vi "map_XY_stiffback.vi"() -> ()   [LabVIEW 2011]
panel:
  in  "KILL":bool
  in  "PAUSE":bool
  in  "RESUME":bool
  in  "QUIT":bool
  in  "up done":bool
  in  "z up":bool
  in  "Done":bool
  in  "z go to table 2":bool
  in  "z go to table":bool
  in  "go to y pos":bool
  in  "goto x pos":bool
  in  "End":bool
  in  "zero z - end":bool
  in  "zero x - end":bool
  in  "zero y - end":bool
  in  "goto z pos":bool
  in  "positioning done":bool
  out "output":string
  out "command":string
  in  "zero done":bool
  in  "zero z":bool
  in  "zero x":bool
  in  "zero y":bool
  # "Comandi di emergenza"
  # "MAPPING XY STIFFBACK"
  # "Posiziono in zero"
  # "Vado sulla piastra \ne azzero"
  # "Alzo il comparatore"
  # "Vado in posizione"
  # "Ritorno a zero"
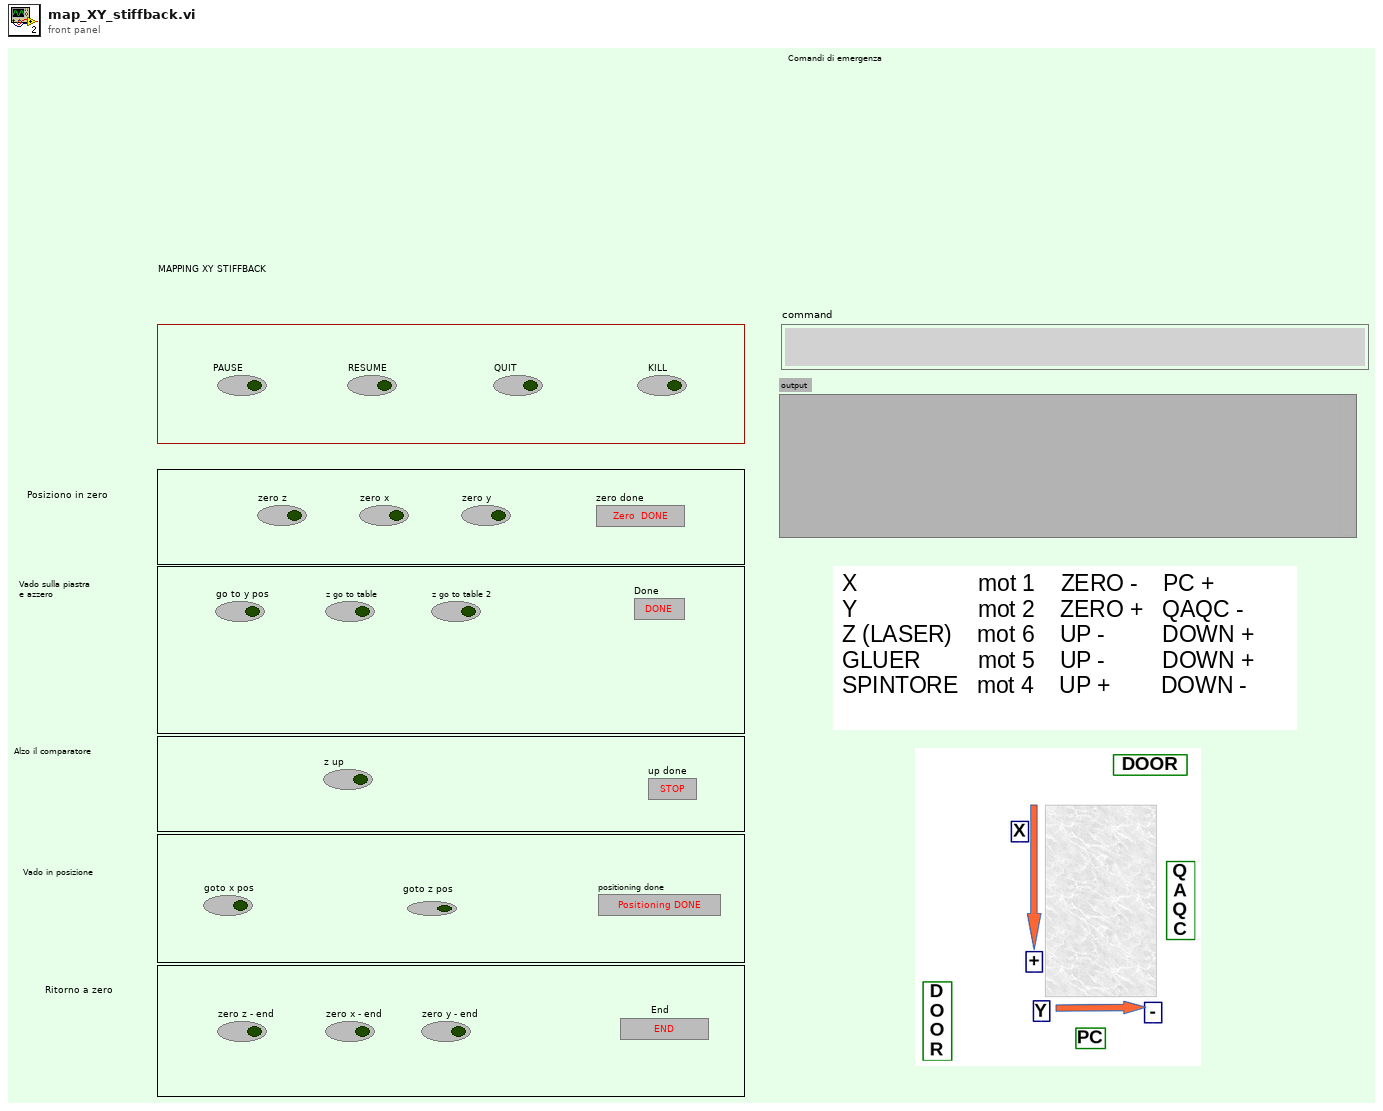
[diagram p1: front panel]
types:
  T1 = enum16{"open", "replace", "create", "open or create", "replace or create", "replace or create with confirmation"}
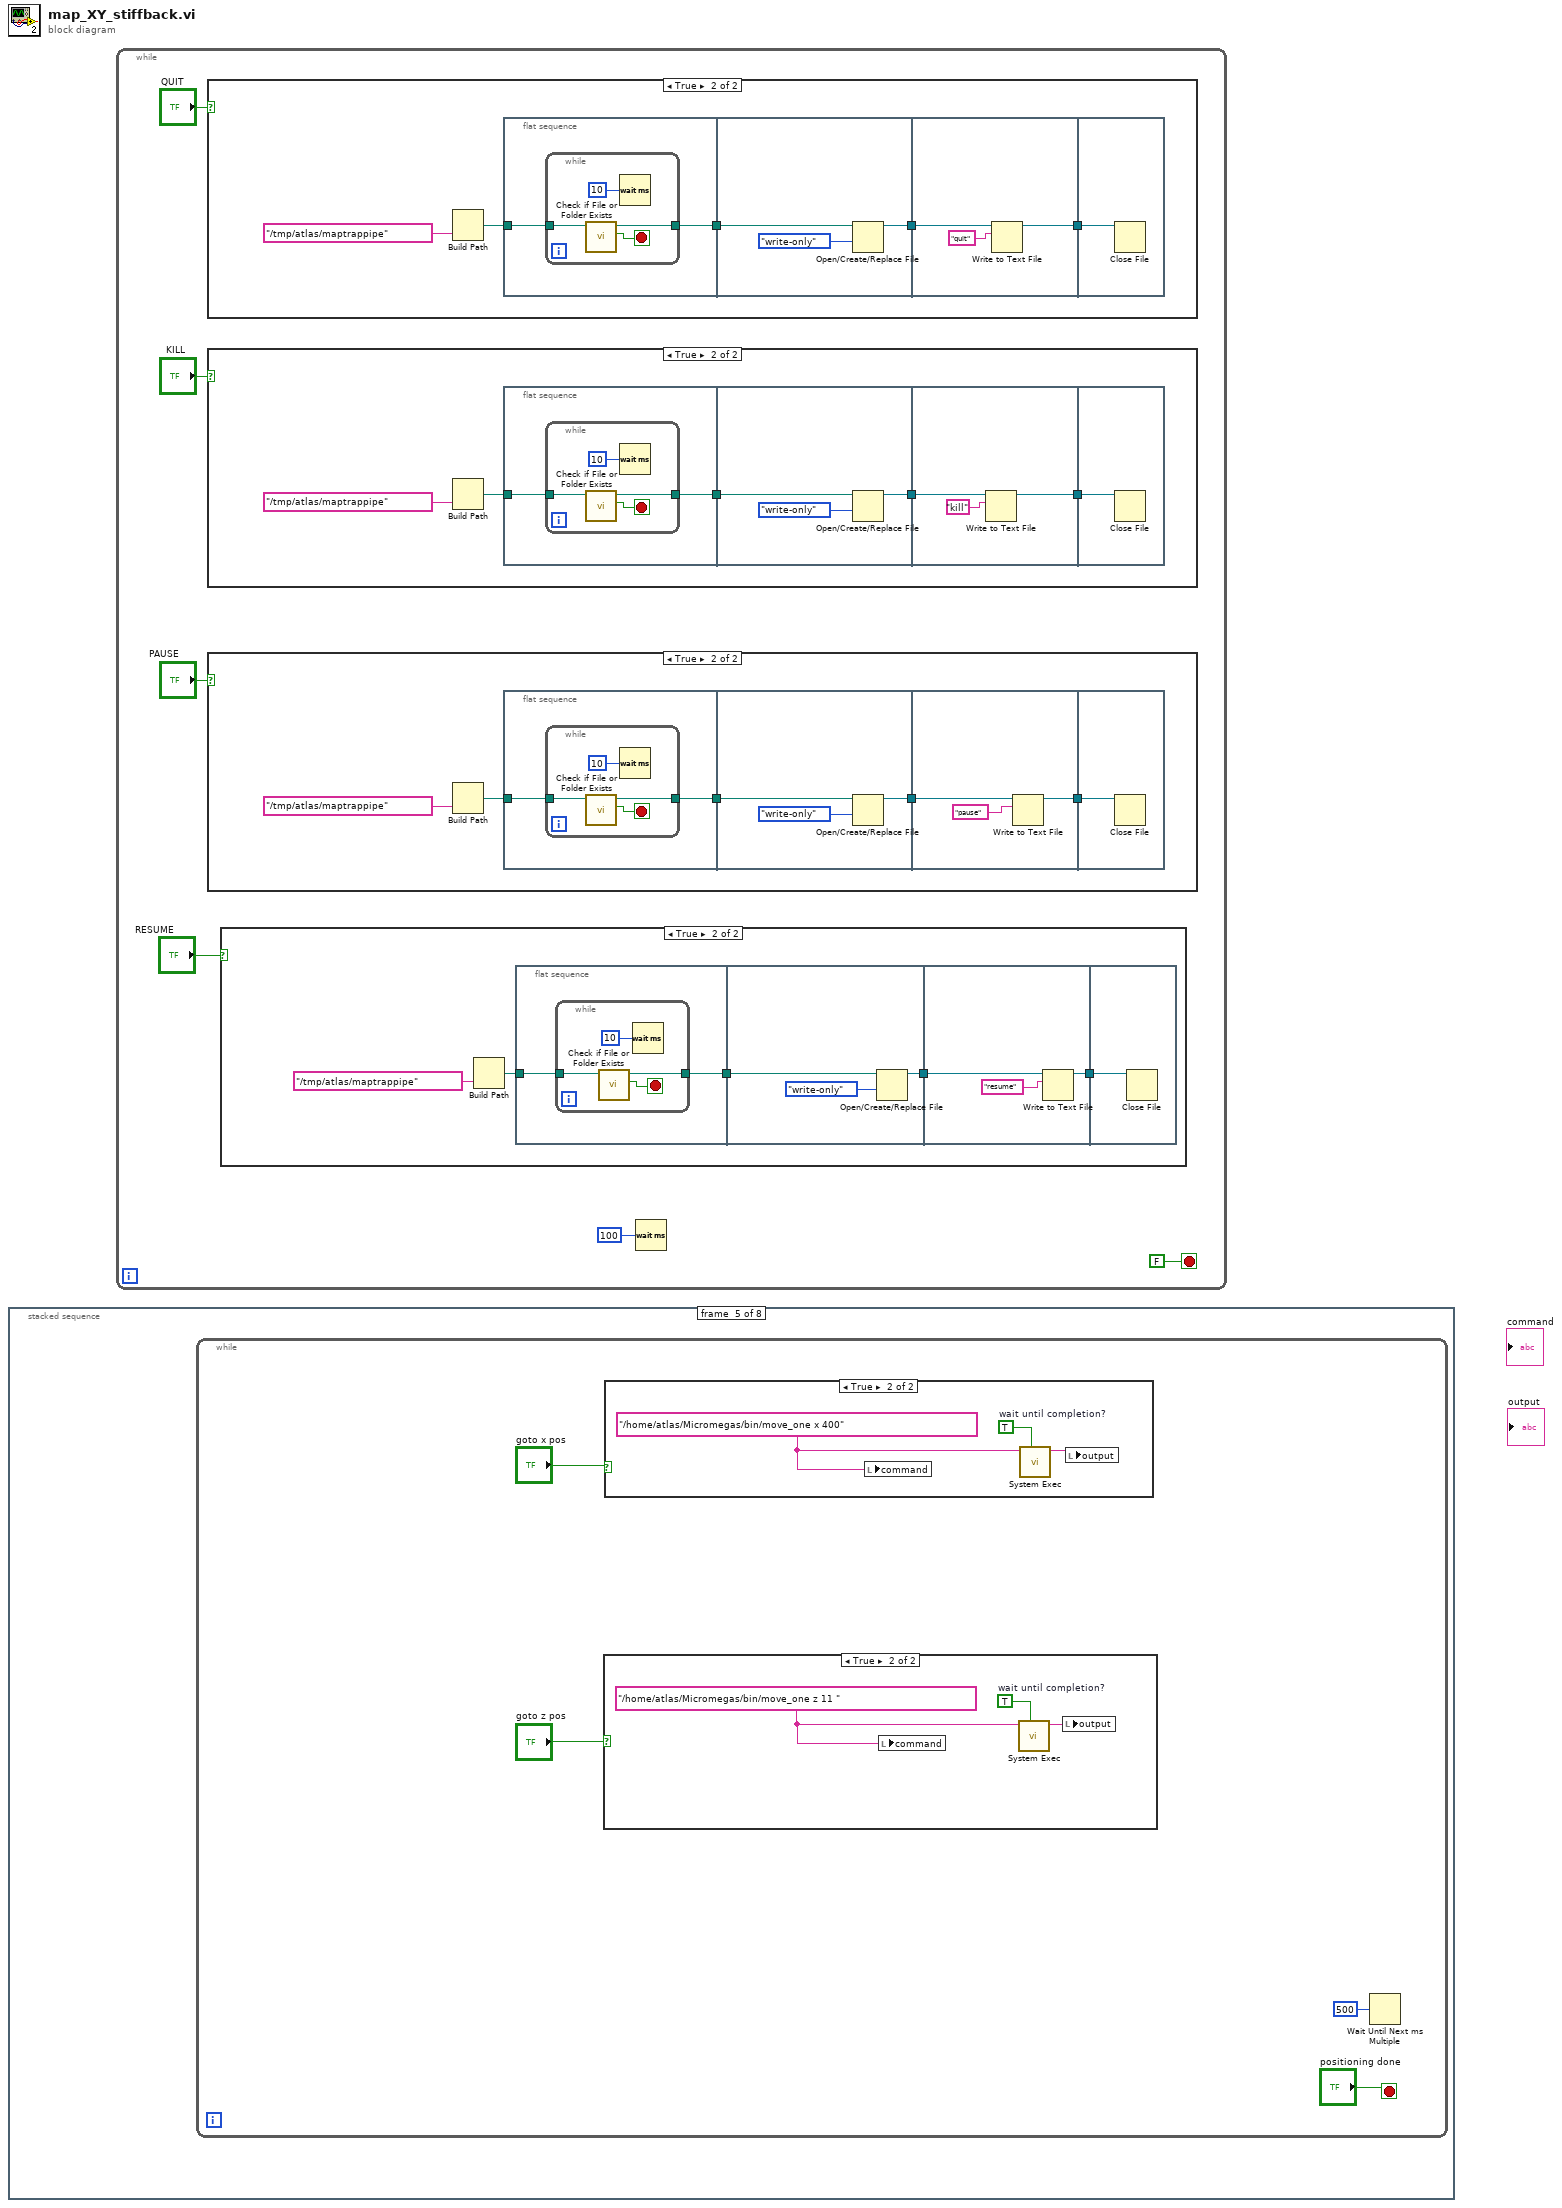
[diagram p0: block diagram]
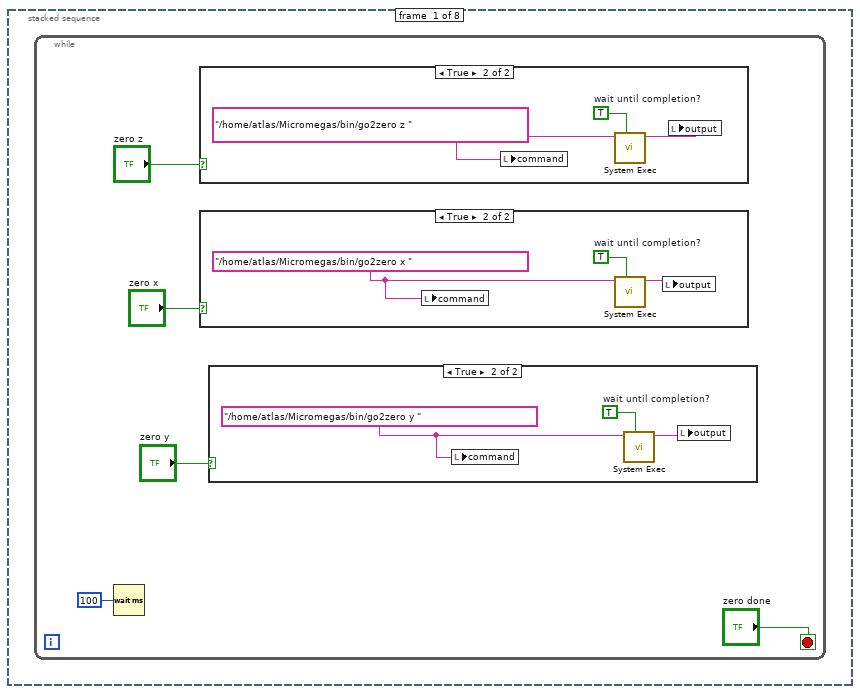
[diagram p6: hidden frame]
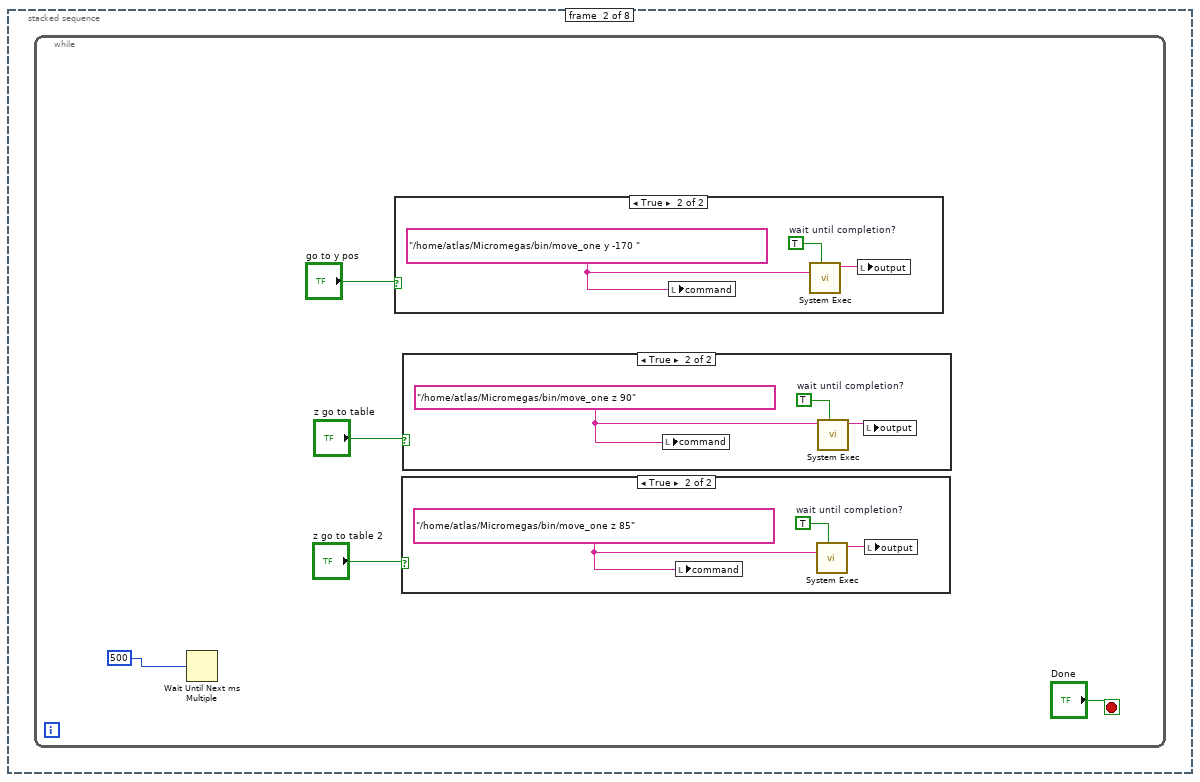
[diagram p10: hidden frame]
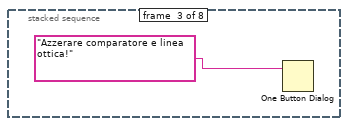
[diagram p14: hidden frame]
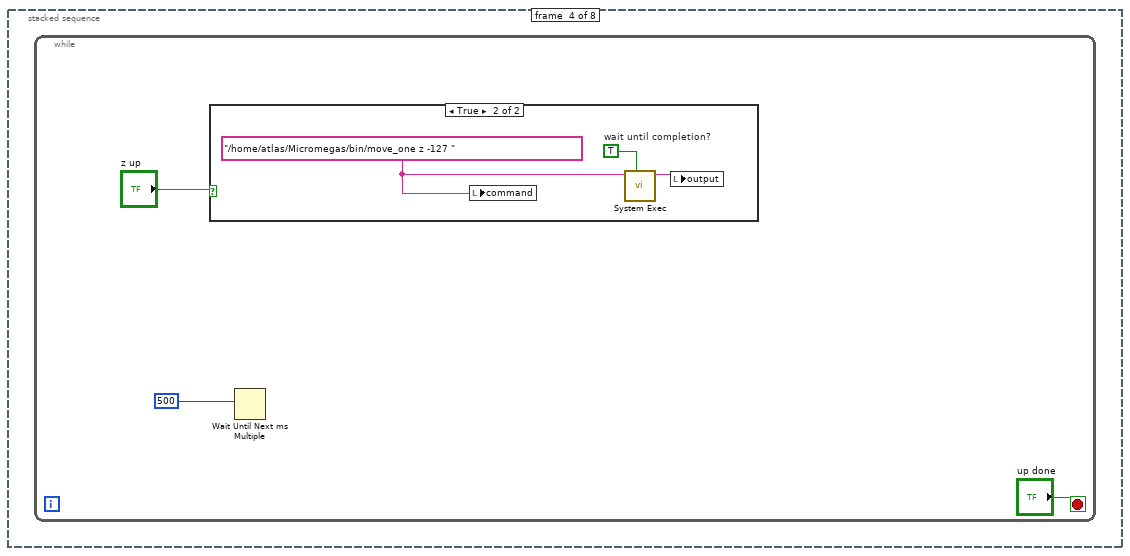
[diagram p15: hidden frame]
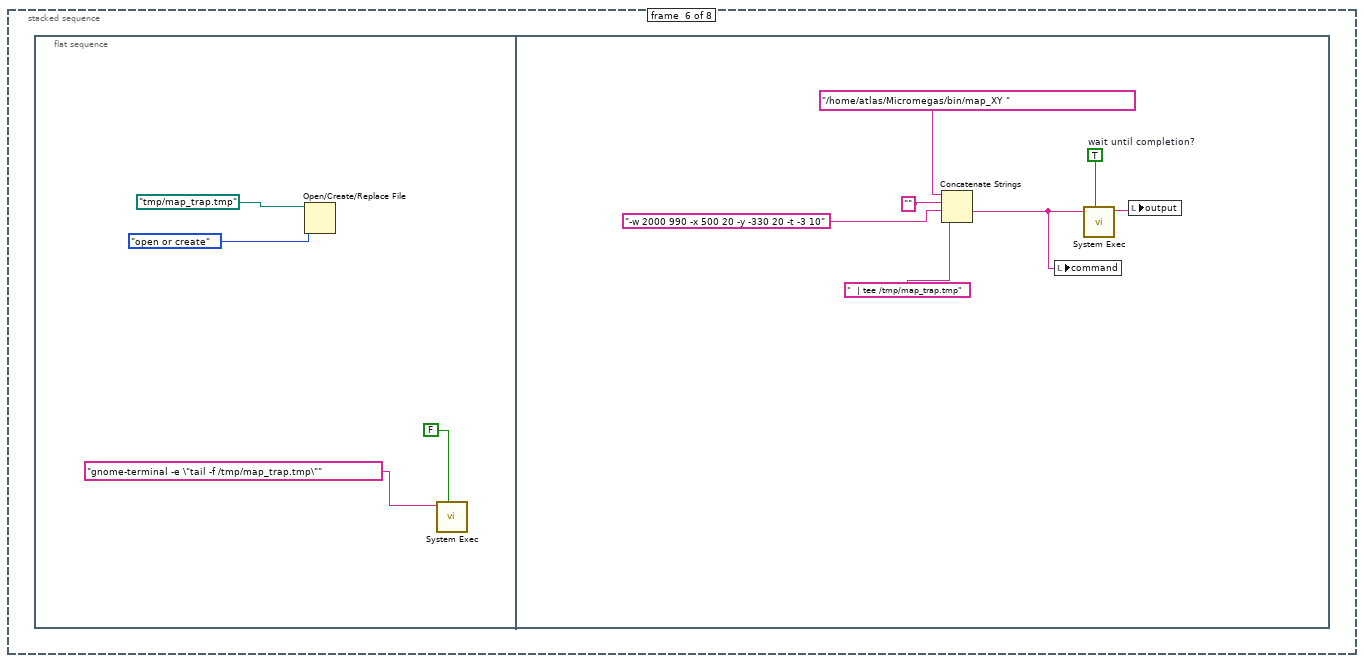
[diagram p19: hidden frame]
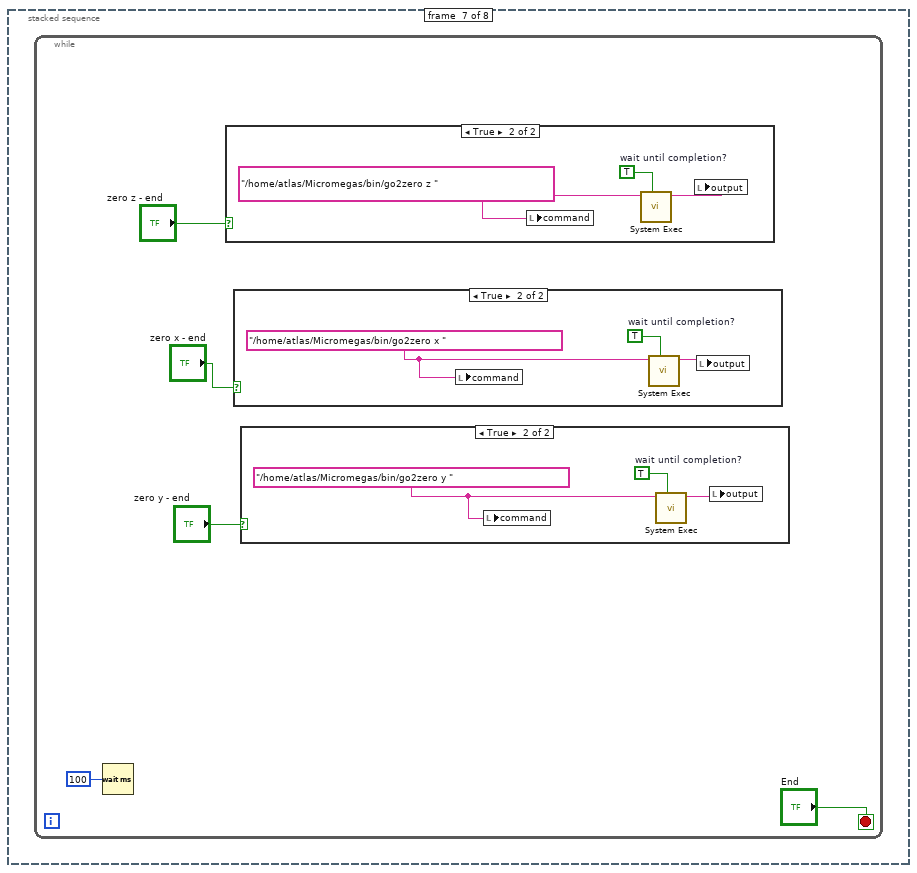
[diagram p20: hidden frame]
diagram:
  n1 = stacked-sequence {
    frame #0 {
      n2 = while {
        stop <- "zero done" stop-if-true
        n3 = Wait (ms)(milliseconds to wait=u32 100) -> ()  [unwired: 1 out]
        n4 = case shown="True" "zero z" {
          frame False {
          }
          frame True {
            w13 = "/home/atlas/Micromegas/bin/go2zero z " ("string")
            w14 = TRUE  # wait until completion?
            n5 = local write "command"(w13) -> ()
            n6 = call <vilib>:"System Exec.vi"("wait until completion? (T)"=w14, "command line"=w13) -> ("standard output"=w12:string)  [unwired: 6 in, 3 out]
            n7 = local write "output"(w12) -> ()
          }
        }
        n8 = case shown="True" "zero x" {
          frame False {
          }
          frame True {
            w10 = "/home/atlas/Micromegas/bin/go2zero x " ("string")
            w11 = TRUE  # wait until completion?
            n9 = local write "command"(w10) -> ()
            n10 = call <vilib>:"System Exec.vi"("wait until completion? (T)"=w11, "command line"=w10) -> ("standard output"=w9:string)  [unwired: 6 in, 3 out]
            n11 = local write "output"(w9) -> ()
          }
        }
        n12 = case shown="True" "zero y" {
          frame False {
          }
          frame True {
            w7 = "/home/atlas/Micromegas/bin/go2zero y " ("string")
            w8 = TRUE  # wait until completion?
            n13 = local write "command"(w7) -> ()
            n14 = call <vilib>:"System Exec.vi"("wait until completion? (T)"=w8, "command line"=w7) -> ("standard output"=w6:string)  [unwired: 6 in, 3 out]
            n15 = local write "output"(w6) -> ()
          }
        }
      }
    }
    frame #1 {
      n16 = while {
        stop <- "Done" stop-if-true
        n17 = Wait Until Next ms Multiple(millisecond multiple=u32 500 ("millisecond timer value")) -> ()  [unwired: 1 out]
        n18 = case shown="True" "go to y pos" {
          frame False {
          }
          frame True {
            w26 = "/home/atlas/Micromegas/bin/move_one y -170 " ("string")
            w28 = TRUE  # wait until completion?
            n19 = local write "command"(w26) -> ()
            n20 = call <vilib>:"System Exec.vi"("wait until completion? (T)"=w28, "command line"=w26) -> ("standard output"=w27:string)  [unwired: 6 in, 3 out]
            n21 = local write "output"(w27) -> ()
          }
        }
        n22 = case shown="True" "z go to table 2" {
          frame False {
          }
          frame True {
            w20 = "/home/atlas/Micromegas/bin/move_one z 85" ("string")
            w22 = TRUE  # wait until completion?
            n23 = local write "command"(w20) -> ()
            n24 = call <vilib>:"System Exec.vi"("wait until completion? (T)"=w22, "command line"=w20) -> ("standard output"=w21:string)  [unwired: 6 in, 3 out]
            n25 = local write "output"(w21) -> ()
          }
        }
        n26 = case shown="True" "z go to table" {
          frame False {
          }
          frame True {
            w23 = "/home/atlas/Micromegas/bin/move_one z 90" ("string")
            w25 = TRUE  # wait until completion?
            n27 = local write "command"(w23) -> ()
            n28 = call <vilib>:"System Exec.vi"("wait until completion? (T)"=w25, "command line"=w23) -> ("standard output"=w24:string)  [unwired: 6 in, 3 out]
            n29 = local write "output"(w24) -> ()
          }
        }
      }
    }
    frame #2 {
      n30 = One Button Dialog(message="Azzerare comparatore e linea ottica!") -> ()  [unwired: 1 in, 1 out]
    }
    frame #3 {
      n31 = while {
        stop <- "up done" stop-if-true
        n32 = case shown="True" "z up" {
          frame False {
          }
          frame True {
            w33 = "/home/atlas/Micromegas/bin/move_one z -127 " ("string")
            w35 = TRUE  # wait until completion?
            n33 = local write "command"(w33) -> ()
            n34 = call <vilib>:"System Exec.vi"("wait until completion? (T)"=w35, "command line"=w33) -> ("standard output"=w34:string)  [unwired: 6 in, 3 out]
            n35 = local write "output"(w34) -> ()
          }
        }
        n36 = Wait Until Next ms Multiple(millisecond multiple=u32 500 ("millisecond timer value")) -> ()  [unwired: 1 out]
      }
    }
    frame #4 {
      n37 = while {
        stop <- "positioning done" stop-if-true
        n38 = case shown="True" "goto z pos" {
          frame False {
          }
          frame True {
            w40 = "/home/atlas/Micromegas/bin/move_one z 11 " ("string")
            w42 = TRUE  # wait until completion?
            n39 = local write "command"(w40) -> ()
            n40 = call <vilib>:"System Exec.vi"("wait until completion? (T)"=w42, "command line"=w40) -> ("standard output"=w41:string)  [unwired: 6 in, 3 out]
            n41 = local write "output"(w41) -> ()
          }
        }
        n42 = case shown="True" "goto x pos" {
          frame False {
          }
          frame True {
            w43 = "/home/atlas/Micromegas/bin/move_one x 400" ("string")
            w45 = TRUE  # wait until completion?
            n43 = local write "command"(w43) -> ()
            n44 = call <vilib>:"System Exec.vi"("wait until completion? (T)"=w45, "command line"=w43) -> ("standard output"=w44:string)  [unwired: 6 in, 3 out]
            n45 = local write "output"(w44) -> ()
          }
        }
        n46 = Wait Until Next ms Multiple(millisecond multiple=u32 500) -> ()  [unwired: 1 out]
      }
    }
    frame #5 {
      n47 = flat-sequence {
        frame #0 {
          n48 = Open/Create/Replace File(file path (use dialog)=path "/tmp/map_trap.tmp", operation (0:open)=T1."open or create") -> ()  [unwired: 4 in, 3 out]
          n49 = call <vilib>:"System Exec.vi"("wait until completion? (T)"=FALSE, "command line"="gnome-terminal -e \"tail -f /tmp/map_trap.tmp\"") -> ()  [unwired: 6 in, 4 out]
        }
        frame #1 {
          w56 = TRUE  # wait until completion?
          n50 = Concatenate Strings("/home/atlas/Micromegas/bin/map_XY " ("string"), "" ("string"), "-w 2000 990 -x 500 20 -y -330 20 -t -3 10" ("string"), "  | tee /tmp/map_trap.tmp" ("string")) -> (w51:string)
          n51 = local write "command"(w51) -> ()
          n52 = call <vilib>:"System Exec.vi"("wait until completion? (T)"=w56, "command line"=w51) -> ("standard output"=w50:string)  [unwired: 6 in, 3 out]
          n53 = local write "output"(w50) -> ()
        }
      }
    }
    frame #6 {
      n54 = while {
        stop <- "End" stop-if-true
        n55 = Wait (ms)(milliseconds to wait=u32 100) -> ()  [unwired: 1 out]
        n56 = case shown="True" "zero z - end" {
          frame False {
          }
          frame True {
            w69 = "/home/atlas/Micromegas/bin/go2zero z " ("string")
            w70 = TRUE  # wait until completion?
            n57 = local write "command"(w69) -> ()
            n58 = call <vilib>:"System Exec.vi"("wait until completion? (T)"=w70, "command line"=w69) -> ("standard output"=w68:string)  [unwired: 6 in, 3 out]
            n59 = local write "output"(w68) -> ()
          }
        }
        n60 = case shown="True" "zero x - end" {
          frame False {
          }
          frame True {
            w66 = "/home/atlas/Micromegas/bin/go2zero x " ("string")
            w67 = TRUE  # wait until completion?
            n61 = local write "command"(w66) -> ()
            n62 = call <vilib>:"System Exec.vi"("wait until completion? (T)"=w67, "command line"=w66) -> ("standard output"=w65:string)  [unwired: 6 in, 3 out]
            n63 = local write "output"(w65) -> ()
          }
        }
        n64 = case shown="True" "zero y - end" {
          frame False {
          }
          frame True {
            w63 = "/home/atlas/Micromegas/bin/go2zero y " ("string")
            w64 = TRUE  # wait until completion?
            n65 = local write "command"(w63) -> ()
            n66 = call <vilib>:"System Exec.vi"("wait until completion? (T)"=w64, "command line"=w63) -> ("standard output"=w62:string)  [unwired: 6 in, 3 out]
            n67 = local write "output"(w62) -> ()
          }
        }
      }
    }
    frame #7 {
      n68 = One Button Dialog(message="Per comodita`, rinominare il file (non verra` comunque sovrascritto)") -> ()  [unwired: 1 in, 1 out]
    }
  }
  n69 = while {
    stop <- FALSE stop-if-true
    n70 = case shown="True" "QUIT" {
      frame False {
      }
      frame True {
        n71 = Build Path(name or relative path="/tmp/atlas/maptrappipe" ("string")) -> (appended path=w132:path)  [unwired: 1 in]
        n72 = flat-sequence {
          tunnel: [w138] -> w136
          tunnel: w132 -> [w137]
          tunnel: w136 -> [w145]
          tunnel: [w143] -> w135
          tunnel: w135 -> [w148]
          tunnel: [w147] -> w134
          tunnel: w134 -> [w149]
          frame #0 {
            n73 = while {
              tunnel: [w140] -> w138
              tunnel: w137 -> [w139]
              stop <- w141 stop-if-true
              n74 = call <vilib>:"Check if File or Folder Exists.vi"("path"=w139) -> ("file or folder exists?"=w141:bool, "dup path"=w140:path)  [unwired: 8 in, 1 out]
              n75 = Wait (ms)(milliseconds to wait=u32 10) -> ()  [unwired: 1 out]
            }
          }
          frame #1 {
            n76 = Open/Create/Replace File(file path (use dialog)=w145, access (0:read/write)=enum16{"read/write", "read-only", "write-only"}."write-only") -> (refnum out=w143:refnum<file>)  [unwired: 4 in, 2 out]
          }
          frame #2 {
            n77 = Write to Text File(file (use dialog)=w148, text="quit") -> (refnum out=w147:refnum<file>)  [unwired: 2 in, 2 out]
          }
          frame #3 {
            n78 = Close File(refnum=w149) -> ()  [unwired: 1 in, 2 out]
          }
        }
      }
    }
    n79 = case shown="True" "KILL" {
      frame False {
      }
      frame True {
        n80 = Build Path(name or relative path="/tmp/atlas/maptrappipe" ("string")) -> (appended path=w96:path)  [unwired: 1 in]
        n81 = flat-sequence {
          tunnel: [w102] -> w100
          tunnel: w96 -> [w101]
          tunnel: w100 -> [w109]
          tunnel: [w107] -> w99
          tunnel: w99 -> [w112]
          tunnel: [w111] -> w98
          tunnel: w98 -> [w113]
          frame #0 {
            n82 = while {
              tunnel: [w104] -> w102
              tunnel: w101 -> [w103]
              stop <- w105 stop-if-true
              n83 = call <vilib>:"Check if File or Folder Exists.vi"("path"=w103) -> ("file or folder exists?"=w105:bool, "dup path"=w104:path)  [unwired: 8 in, 1 out]
              n84 = Wait (ms)(milliseconds to wait=u32 10) -> ()  [unwired: 1 out]
            }
          }
          frame #1 {
            n85 = Open/Create/Replace File(file path (use dialog)=w109, access (0:read/write)=enum16{"read/write", "read-only", "write-only"}."write-only") -> (refnum out=w107:refnum<file>)  [unwired: 4 in, 2 out]
          }
          frame #2 {
            n86 = Write to Text File(file (use dialog)=w112, text="kill") -> (refnum out=w111:refnum<file>)  [unwired: 2 in, 2 out]
          }
          frame #3 {
            n87 = Close File(refnum=w113) -> ()  [unwired: 1 in, 2 out]
          }
        }
      }
    }
    n88 = case shown="True" "PAUSE" {
      frame False {
      }
      frame True {
        n89 = Build Path(name or relative path="/tmp/atlas/maptrappipe" ("string")) -> (appended path=w78:path)  [unwired: 1 in]
        n90 = flat-sequence {
          tunnel: [w84] -> w82
          tunnel: w78 -> [w83]
          tunnel: w82 -> [w91]
          tunnel: [w89] -> w81
          tunnel: w81 -> [w94]
          tunnel: [w93] -> w80
          tunnel: w80 -> [w95]
          frame #0 {
            n91 = while {
              tunnel: [w86] -> w84
              tunnel: w83 -> [w85]
              stop <- w87 stop-if-true
              n92 = call <vilib>:"Check if File or Folder Exists.vi"("path"=w85) -> ("file or folder exists?"=w87:bool, "dup path"=w86:path)  [unwired: 8 in, 1 out]
              n93 = Wait (ms)(milliseconds to wait=u32 10) -> ()  [unwired: 1 out]
            }
          }
          frame #1 {
            n94 = Open/Create/Replace File(file path (use dialog)=w91, access (0:read/write)=enum16{"read/write", "read-only", "write-only"}."write-only") -> (refnum out=w89:refnum<file>)  [unwired: 4 in, 2 out]
          }
          frame #2 {
            n95 = Write to Text File(file (use dialog)=w94, text="pause") -> (refnum out=w93:refnum<file>)  [unwired: 2 in, 2 out]
          }
          frame #3 {
            n96 = Close File(refnum=w95) -> ()  [unwired: 1 in, 2 out]
          }
        }
      }
    }
    n97 = case shown="True" "RESUME" {
      frame False {
      }
      frame True {
        n98 = Build Path(name or relative path="/tmp/atlas/maptrappipe" ("string")) -> (appended path=w114:path)  [unwired: 1 in]
        n99 = flat-sequence {
          tunnel: [w120] -> w118
          tunnel: w114 -> [w119]
          tunnel: w118 -> [w127]
          tunnel: [w125] -> w117
          tunnel: w117 -> [w130]
          tunnel: [w129] -> w116
          tunnel: w116 -> [w131]
          frame #0 {
            n100 = while {
              tunnel: [w122] -> w120
              tunnel: w119 -> [w121]
              stop <- w123 stop-if-true
              n101 = call <vilib>:"Check if File or Folder Exists.vi"("path"=w121) -> ("file or folder exists?"=w123:bool, "dup path"=w122:path)  [unwired: 8 in, 1 out]
              n102 = Wait (ms)(milliseconds to wait=u32 10) -> ()  [unwired: 1 out]
            }
          }
          frame #1 {
            n103 = Open/Create/Replace File(file path (use dialog)=w127, access (0:read/write)=enum16{"read/write", "read-only", "write-only"}."write-only") -> (refnum out=w125:refnum<file>)  [unwired: 4 in, 2 out]
          }
          frame #2 {
            n104 = Write to Text File(file (use dialog)=w130, text="resume") -> (refnum out=w129:refnum<file>)  [unwired: 2 in, 2 out]
          }
          frame #3 {
            n105 = Close File(refnum=w131) -> ()  [unwired: 1 in, 2 out]
          }
        }
      }
    }
    n106 = Wait (ms)(milliseconds to wait=100) -> ()  [unwired: 1 out]
  }
